vi "Autonomous Independent.vi"   [LabVIEW 2015]
doc: "This VI is called when autonomous begins, and will automatically be terminated when autonomous ends. You can carry out timed or sensor driven robot movement independently without needing to return to the caller."
uses:
  <vilib>/Rock Robotics/WPI/Utilities/WPI_GetSetVariantRefNum.vi
  <vilib>/Rock Robotics/Network Tables/NT Read String.vi
  <vilib>/Rock Robotics/Network Tables/NT Write Numeric Array.vi
  <vilib>/Rock Robotics/Network Tables/NT Read Number.vi
  <vilib>/Rock Robotics/WPI/RobotDrive/WPI_RobotDriveArcadeDrive_Standard(NoSaturation).vi
  <vilib>/Rock Robotics/WPI/RobotDrive/WPI_RobotDriveSafetyCheck.vi
panel:
  # "Be sure to right-click and choose Data Operations>>Make Current Value default if you want to save the array values with the VI"
types:
  T1 = typedef "WPI_JoystickDevRef.ctl" = cluster{"Device":T2}
  T2 = typedef "WPI_JoystickDeviceEnum.ctl" = enum16{"USB 0", "USB 1", "USB 2", "USB 3", "USB 4", "USB 5"}
  T3 = typedef "WPI_RobotDriveDevRef.ctl" = cluster{"DevStatus":errorcluster, "Motors[]":T4[], "Square Inputs":bool, "Max Output":dbl}
  T4 = typedef "WPI_MotorControlDeviceRef.ctl" = cluster{"DeviceStatus":errorcluster, "Type":T5, "PWM":cluster{"PWM Channel":T6, "DeadBand":T7}, "CAN":cluster{"Device Number":u8, "Control Mode":T8, "Semaphore":T9, "Max Vout":dbl, "TalonSRX Control Mode":T10}, "Invert":bool}
  T5 = typedef "WPI_MotorControlType.ctl" = enum16{"PWM", "CAN", "CANTalonSRX"}
  T6 = typedef "FPGA_DIOPWMChannel.ctl" = enum8{"PWM 0", "PWM 1", "PWM 2", "PWM 3", "PWM 4", "PWM 5", "PWM 6", "PWM 7", "PWM 8", "PWM 9", "PWM MXP 0", "PWM MXP 1", "PWM MXP 2", "PWM MXP 3", "PWM MXP 4", "PWM MXP 5", "PWM MXP 6", "PWM MXP 7", "PWM MXP 8", "PWM MXP 9", "Invalid"}
  T7 = typedef "WPI_PWMDeadband.ctl" = cluster{"Name":string, "maxPositivePwm":i32, "minPositivePwm":i32, "centerPwm":i32, "maxNegativePwm":i32, "minNegativePwm":i32, "angularRange":u16}
  T8 = typedef "WPI_CANJaguar_ControlMode.ctl" = enum8{"Percent VBus", "Current", "Speed", "Position", "Voltage"}
  T9 = typedef "Semaphore RefNum" = refnum<k1>
  T10 = typedef "WPI_CANTalonSRX_APIControlMode.ctl" = enum8{"Percent VBus", "Speed", "Position", "Slave", "Unchanged / Invalid", "Voltage Compensation", "Current", "Motion Profile"}
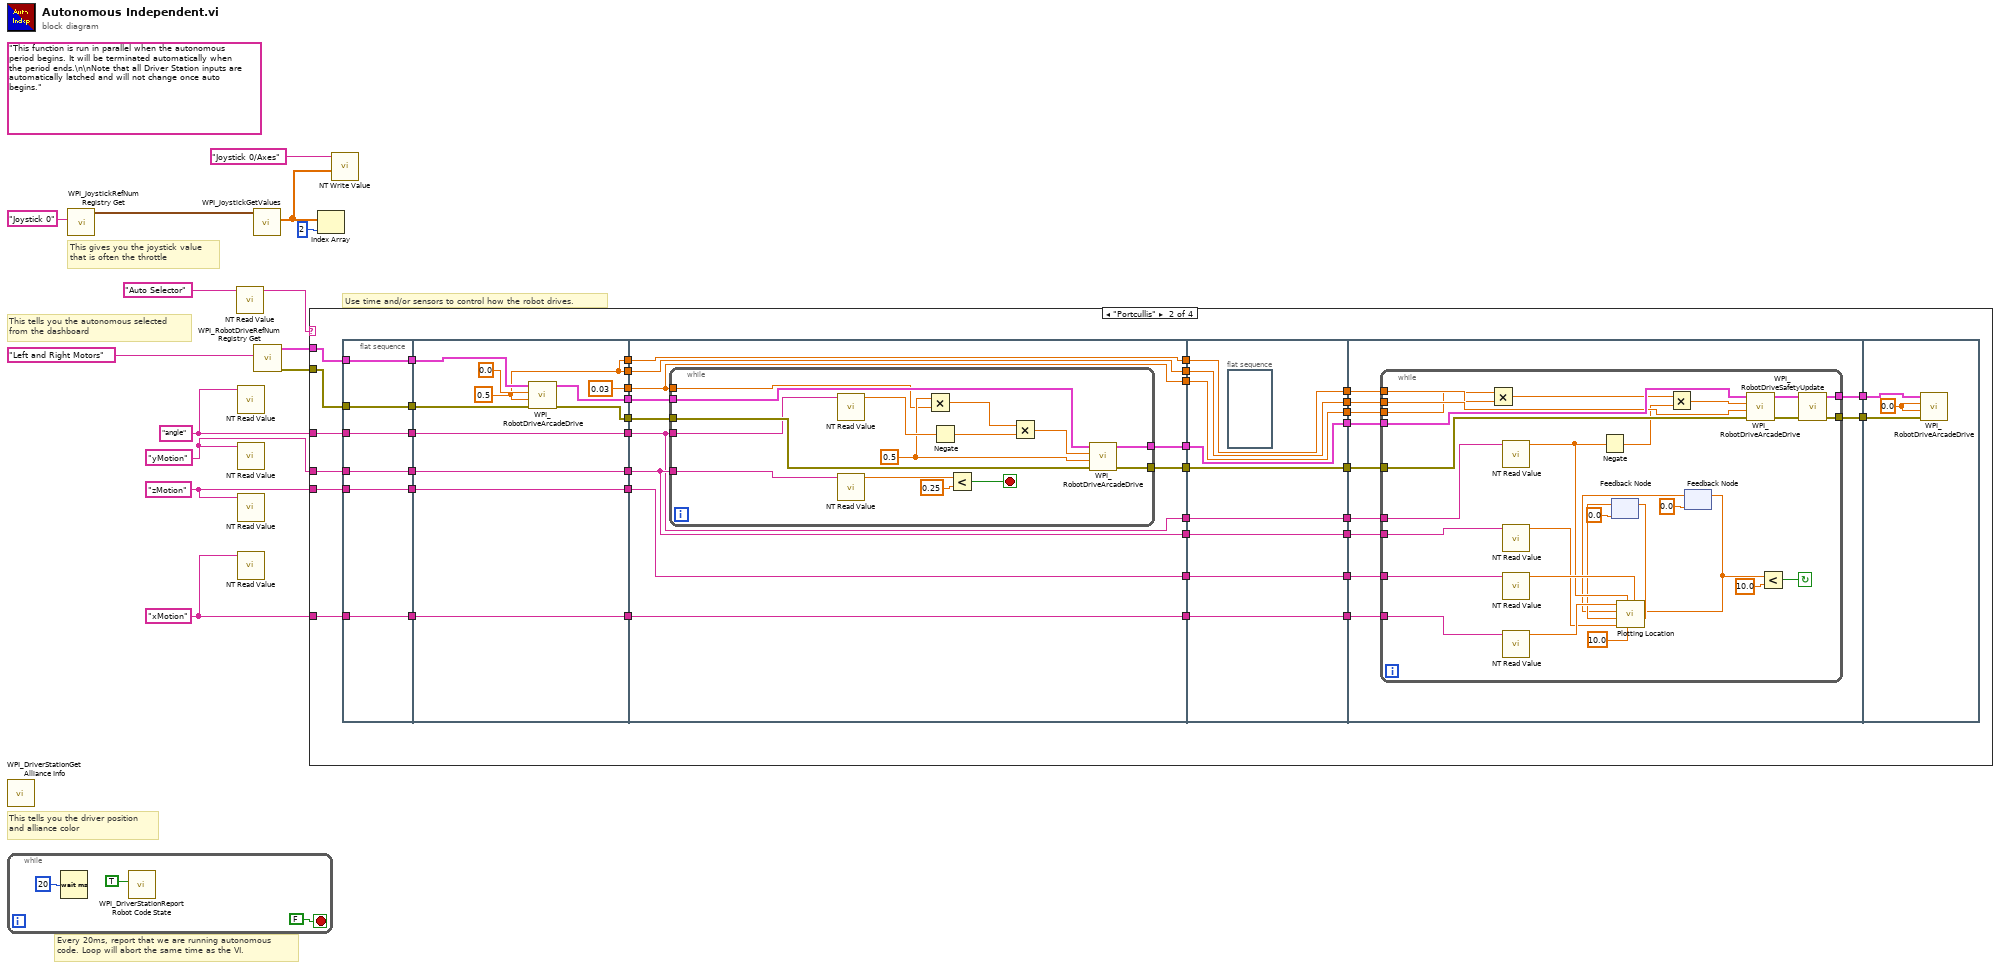
[diagram p0: block diagram]
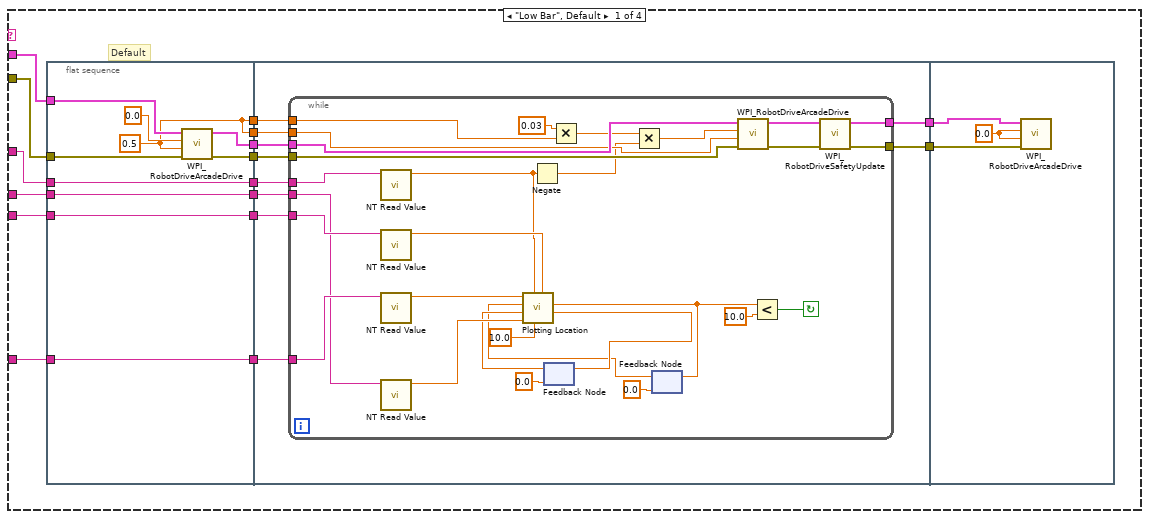
[diagram p2: hidden frame]
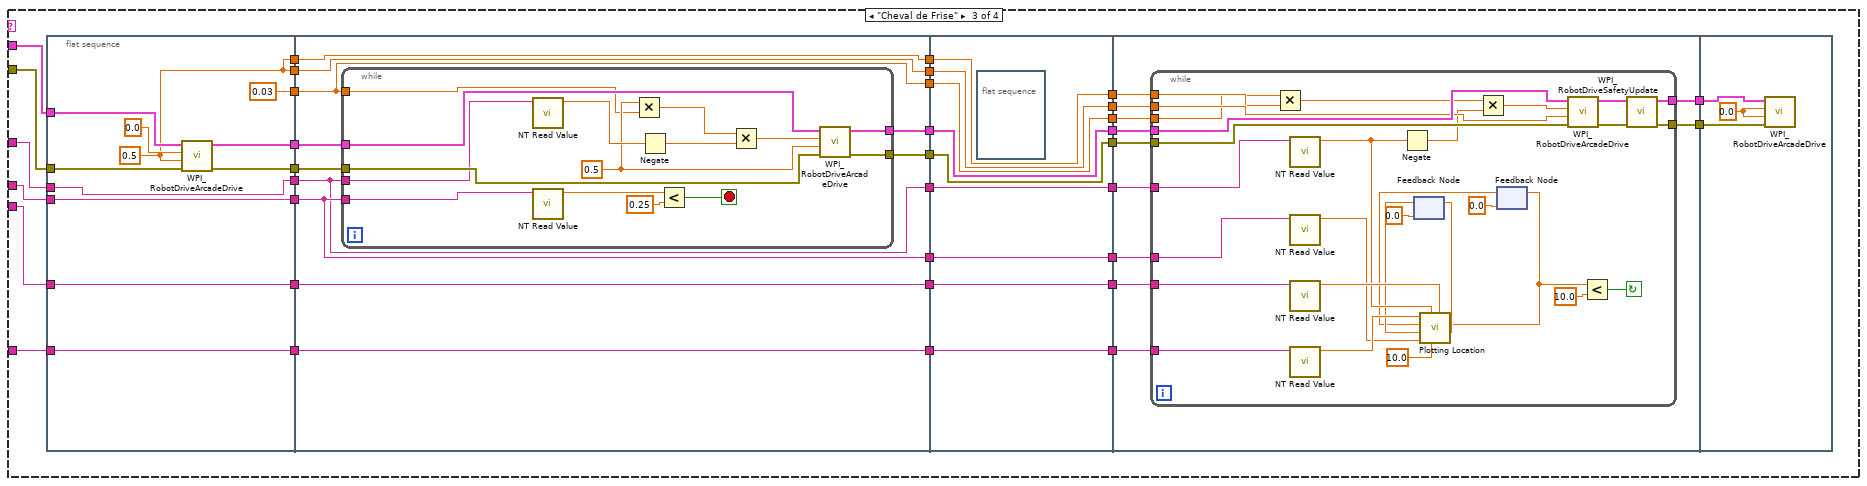
[diagram p3: hidden frame]
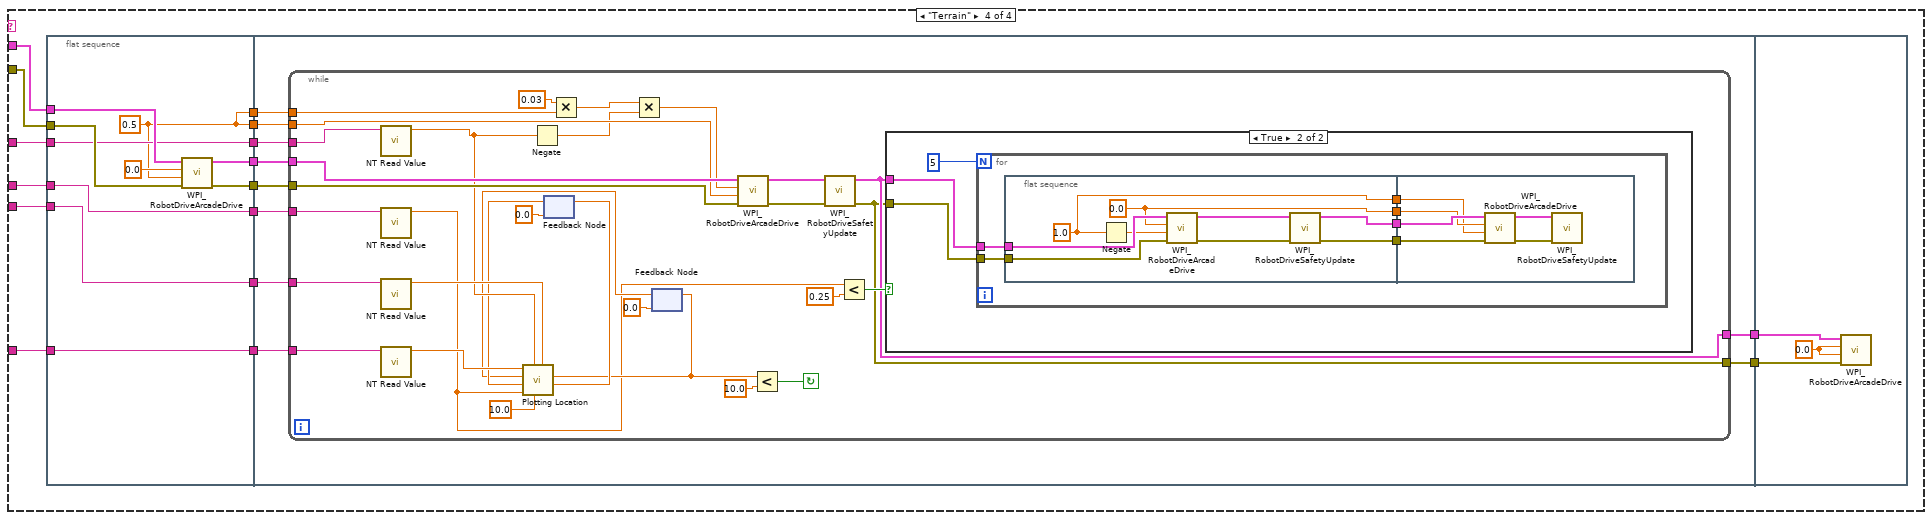
[diagram p4: hidden frame]
diagram:
  w4 = "angle" ("Name")
  w1 = "yMotion" ("Name")
  w2 = "zMotion" ("Name")
  w3 = "xMotion" ("Name")
  (unwired) "This function is run in parallel when the autonomous period begins. It will be terminated automatically when the period ends.\n\nNote that all Driver Station inputs are automatically latched and will not change once auto begins."
  # "This tells you the autonomous selected\nfrom the dashboard"
  # "Every 20ms, report that we are running autonomous\ncode. Loop will abort the same time as the VI."
  # "This gives you the joystick value\nthat is often the throttle"
  # "Use time and/or sensors to control how the robot drives."
  # "This tells you the driver position\nand alliance color"
  n1 = call <vilib>:"WPI_DriverStationGet Alliance Info.vi"() -> ()  [unwired: 12 out]
  n2 = while {
    stop <- FALSE stop-if-true
    n3 = Wait (ms)(milliseconds to wait=u32 20) -> ()  [unwired: 1 out]
    n4 = call <vilib>:"WPI_DriverStationReport Robot Code State.vi"("Autonomous"=TRUE) -> ()  [unwired: 10 in, 1 out]
  }
  n5 = call <vilib>:"WPI_JoystickRefNum Registry Get.vi"("refnum name"="Joystick 0") -> ("JoystickDevRef"=w13:T1)  [unwired: 1 in, 9 out]
  n6 = call-poly <vilib>:"NT Read Value.vi"("Name"="Auto Selector") -> ("String"=w10:string)  [unwired: 9 in, 1 out]
  n7 = call-poly <vilib>:"NT Read Value.vi"("Name"=w4) -> ()  [unwired: 9 in, 2 out]
  n8 = call-poly <vilib>:"NT Read Value.vi"("Name"=w1) -> ()  [unwired: 9 in, 2 out]
  n9 = call-poly <vilib>:"NT Read Value.vi"("Name"=w2) -> ()  [unwired: 9 in, 2 out]
  n10 = call-poly <vilib>:"NT Read Value.vi"("Name"=w3) -> ()  [unwired: 9 in, 2 out]
  n11 = call <vilib>:"WPI_JoystickGetValues.vi"("JoystickDevRef"=w13) -> ("Axes"=w9:dbl[])  [unwired: 6 in, 4 out]
  n12 = call <vilib>:"WPI_RobotDriveRefNum Registry Get.vi"("refnum name"="Left and Right Motors") -> ("error out"=w5:errorcluster, "RobotDriveDevRef"=w6:T3)  [unwired: 9 in]
  n13 = case shown="\"Portcullis\"" w10 {
    tunnel: w6 -> [w33 w124 w223 w351]
    tunnel: w5 -> [w32 w123 w222 w350]
    tunnel: w4 -> [w28 w122 w224 w349]
    tunnel: w3 -> [w26 w120 w227 w346]
    tunnel: w2 -> [w24 w121 w226 w347]
    tunnel: w1 -> [w22 w119 w225 w348]
    frame "Low Bar", Default {
      # "Default"
      n14 = flat-sequence {
        tunnel: w33 -> [w43]
        tunnel: w32 -> [w42]
        tunnel: [w40] -> w31
        tunnel: [w39] -> w30
        tunnel: [w34] -> w29
        tunnel: w28 -> [w38]
        tunnel: [w38] -> w27
        tunnel: w26 -> [w37]
        tunnel: [w37] -> w25
        tunnel: w24 -> [w36]
        tunnel: [w36] -> w23
        tunnel: w22 -> [w35]
        tunnel: [w35] -> w21
        tunnel: [w34] -> w20
        tunnel: w31 -> [w53]
        tunnel: w30 -> [w52]
        tunnel: w29 -> [w51]
        tunnel: w27 -> [w50]
        tunnel: w25 -> [w49]
        tunnel: w23 -> [w48]
        tunnel: w21 -> [w47]
        tunnel: w20 -> [w46]
        tunnel: [w45] -> w19
        tunnel: [w44] -> w18
        tunnel: w19 -> [w85]
        tunnel: w18 -> [w84]
        frame #0 {
          w34 = 0.5 ("Y axis value")
          n15 = call-poly <vilib>:"WPI_RobotDriveArcadeDrive.vi"("error in (no error)"=w42, "Y axis value"=w34, "X axis value"=0.0, "RobotDriveDevRef"=w43) -> ("error out"=w39:errorcluster, "RobotDriveDevRef"=w40:T3)  [unwired: 5 in, 1 out]
        }
        frame #1 {
          n16 = while {
            tunnel: w53 -> [w80]
            tunnel: w52 -> [w79]
            tunnel: w51 -> [w78]
            tunnel: w50 -> [w75]
            tunnel: w49 -> [w74]
            tunnel: w48 -> [w73]
            tunnel: w47 -> [w72]
            tunnel: w46 -> [w70]
            tunnel: [w55] -> w45
            tunnel: [w54] -> w44
            stop <- w63 continue-if-true
            n17 = call-poly <vilib>:"NT Read Value.vi"("Name"=w75) -> ("Numeric"=w65:dbl)  [unwired: 9 in, 1 out]
            n18 = call-poly <vilib>:"NT Read Value.vi"("Name"=w73) -> ("Numeric"=w68:dbl)  [unwired: 9 in, 1 out]
            n19 = call-poly <vilib>:"NT Read Value.vi"("Name"=w74) -> ("Numeric"=w67:dbl)  [unwired: 9 in, 1 out]
            n20 = call-poly <vilib>:"NT Read Value.vi"("Name"=w72) -> ("Numeric"=w66:dbl)  [unwired: 9 in, 1 out]
            n21 = Negate(x=w65) -> (-x=w76:dbl)
            n22 = feedback #1(0.0 ("New Y")) -> (w61:dbl)
            n23 = Multiply(x=0.03, y=w70) -> (x*y=w69:dbl)
            n24 = Multiply(x=w69, y=w76) -> (x*y=w77:dbl)
            n25 = feedback #2(0.0 ("New X")) -> (w58:dbl)
            n26 = call "Plotting Location.vi"("Z Adaption"=w68, "Refresh Rate (ms)"=10.0, "Angle"=w65, "Y-Motion"=w66, "Old Y"=w61, "Old X"=w58, "X-Motion"=w67) -> ("New Y"=w62:dbl, "New X"=w59:dbl)  [unwired: 3 in]
            n27 = feedback-in #1(w62) -> ()
            n28 = feedback-in #2(w59) -> ()
            n29 = call-poly <vilib>:"WPI_RobotDriveArcadeDrive.vi"("error in (no error)"=w79, "Y axis value"=w78, "X axis value"=w77, "RobotDriveDevRef"=w80) -> ("error out"=w81:errorcluster, "RobotDriveDevRef"=w82:T3)  [unwired: 5 in, 1 out]
            n30 = Less?(x=w59, y=10.0) -> (x < y?=w63:bool)
            n31 = call <vilib>:"WPI_RobotDriveSafetyUpdate.vi"("error in (no error)"=w81, "RobotDriveDevRef"=w82) -> ("error out"=w54:errorcluster, "RobotDriveDevRef"=w55:T3)  [unwired: 8 out]
          }
        }
        frame #2 {
          w83 = 0.0 ("X axis value")
          n32 = call-poly <vilib>:"WPI_RobotDriveArcadeDrive.vi"("error in (no error)"=w84, "Y axis value"=w83, "X axis value"=w83, "RobotDriveDevRef"=w85) -> ()  [unwired: 5 in, 3 out]
        }
      }
    }
    frame "Portcullis" {
      n33 = flat-sequence {
        tunnel: w119 -> [w127]
        tunnel: w121 -> [w128]
        tunnel: w120 -> [w129]
        tunnel: w122 -> [w130]
        tunnel: w123 -> [w131]
        tunnel: w124 -> [w132]
        tunnel: [w132] -> w91
        tunnel: [w131] -> w90
        tunnel: [w130] -> w89
        tunnel: [w129] -> w88
        tunnel: [w128] -> w87
        tunnel: [w127] -> w86
        tunnel: [w140] -> w118
        tunnel: [w139] -> w117
        tunnel: [w134] -> w116
        tunnel: [w138] -> w115
        tunnel: [w137] -> w114
        tunnel: [w136] -> w113
        tunnel: [w135] -> w112
        tunnel: [w134] -> w111
        tunnel: [0.03 ("x")] -> w93
        tunnel: w91 -> [w143]
        tunnel: w90 -> [w142]
        tunnel: w89 -> [w138]
        tunnel: w88 -> [w137]
        tunnel: w87 -> [w136]
        tunnel: w86 -> [w135]
        tunnel: w118 -> [w149]
        tunnel: w117 -> [w148]
        tunnel: [w146] -> w109
        tunnel: w116 -> [w154]
        tunnel: [w154] -> w107
        tunnel: w115 -> [w145]
        tunnel: [w145] -> w105
        tunnel: w114 -> [w153]
        tunnel: [w153] -> w103
        tunnel: w113 -> [w152]
        tunnel: [w152] -> w101
        tunnel: w112 -> [w150]
        tunnel: [w150] -> w99
        tunnel: w111 -> [w151]
        tunnel: [w151] -> w97
        tunnel: [w144] -> w94
        tunnel: w93 -> [w144]
        tunnel: [w147] -> w92
        tunnel: [w178] -> w110
        tunnel: w109 -> [w177]
        tunnel: [w177] -> w108
        tunnel: w107 -> [w176]
        tunnel: [w176] -> w106
        tunnel: w105 -> [w175]
        tunnel: [w175] -> w104
        tunnel: w103 -> [w174]
        tunnel: [w174] -> w102
        tunnel: w101 -> [w173]
        tunnel: [w173] -> w100
        tunnel: w99 -> [w172]
        tunnel: [w172] -> w98
        tunnel: w97 -> [w171]
        tunnel: [w171] -> w96
        tunnel: [w170] -> w95
        tunnel: w94 -> [w170]
        tunnel: w92 -> [w178]
        tunnel: w110 -> [w189]
        tunnel: w108 -> [w188]
        tunnel: w106 -> [w187]
        tunnel: w104 -> [w186]
        tunnel: w102 -> [w185]
        tunnel: w100 -> [w184]
        tunnel: w98 -> [w183]
        tunnel: w96 -> [w182]
        tunnel: [w181] -> w126
        tunnel: [w180] -> w125
        tunnel: w95 -> [w179]
        tunnel: w126 -> [w221]
        tunnel: w125 -> [w220]
        frame #0 {
        }
        frame #1 {
          w134 = 0.5 ("Y axis value")
          n34 = call-poly <vilib>:"WPI_RobotDriveArcadeDrive.vi"("error in (no error)"=w142, "Y axis value"=w134, "X axis value"=0.0, "RobotDriveDevRef"=w143) -> ("error out"=w139:errorcluster, "RobotDriveDevRef"=w140:T3)  [unwired: 5 in, 1 out]
        }
        frame #2 {
          n35 = while {
            tunnel: w150 -> [w166]
            tunnel: w149 -> [w165]
            tunnel: w148 -> [w164]
            tunnel: [w163] -> w147
            tunnel: [w162] -> w146
            tunnel: w145 -> [w161]
            tunnel: w144 -> [w156]
            stop <- w167 stop-if-true
            w157 = 0.5 ("Y axis value")
            n36 = call-poly <vilib>:"NT Read Value.vi"("Name"=w161) -> ("Numeric"=w158:dbl)  [unwired: 9 in, 1 out]
            n37 = call-poly <vilib>:"NT Read Value.vi"("Name"=w166) -> ("Numeric"=w169:dbl)  [unwired: 9 in, 1 out]
            n38 = Multiply(x=w157, y=w156) -> (x*y=w159:dbl)
            n39 = Negate(x=w158) -> (-x=w160:dbl)
            n40 = Less?(x=w169, y=0.25) -> (x < y?=w167:bool)
            n41 = Multiply(x=w159, y=w160) -> (x*y=w155:dbl)
            n42 = call-poly <vilib>:"WPI_RobotDriveArcadeDrive.vi"("error in (no error)"=w164, "Y axis value"=w157, "X axis value"=w155, "RobotDriveDevRef"=w165) -> ("error out"=w162:errorcluster, "RobotDriveDevRef"=w163:T3)  [unwired: 5 in, 1 out]
          }
        }
        frame #3 {
          n43 = flat-sequence {
            frame #0 {
            }
          }
        }
        frame #4 {
          n44 = while {
            tunnel: w189 -> [w216]
            tunnel: w188 -> [w215]
            tunnel: w187 -> [w214]
            tunnel: w186 -> [w211]
            tunnel: w185 -> [w210]
            tunnel: w184 -> [w209]
            tunnel: w183 -> [w208]
            tunnel: w182 -> [w207]
            tunnel: [w192] -> w181
            tunnel: [w191] -> w180
            tunnel: w179 -> [w190]
            stop <- w200 continue-if-true
            n45 = Multiply(x=w190, y=w207) -> (x*y=w206:dbl)
            n46 = call-poly <vilib>:"NT Read Value.vi"("Name"=w211) -> ("Numeric"=w202:dbl)  [unwired: 9 in, 1 out]
            n47 = call-poly <vilib>:"NT Read Value.vi"("Name"=w208) -> ("Numeric"=w203:dbl)  [unwired: 9 in, 1 out]
            n48 = call-poly <vilib>:"NT Read Value.vi"("Name"=w209) -> ("Numeric"=w205:dbl)  [unwired: 9 in, 1 out]
            n49 = call-poly <vilib>:"NT Read Value.vi"("Name"=w210) -> ("Numeric"=w204:dbl)  [unwired: 9 in, 1 out]
            n50 = Negate(x=w202) -> (-x=w212:dbl)
            n51 = feedback #3(0.0 ("New Y")) -> (w198:dbl)
            n52 = Multiply(x=w206, y=w212) -> (x*y=w213:dbl)
            n53 = feedback #4(0.0 ("New X")) -> (w195:dbl)
            n54 = call "Plotting Location.vi"("Z Adaption"=w205, "Refresh Rate (ms)"=10.0, "Angle"=w202, "Y-Motion"=w203, "Old Y"=w198, "Old X"=w195, "X-Motion"=w204) -> ("New Y"=w199:dbl, "New X"=w196:dbl)  [unwired: 3 in]
            n55 = feedback-in #3(w199) -> ()
            n56 = feedback-in #4(w196) -> ()
            n57 = call-poly <vilib>:"WPI_RobotDriveArcadeDrive.vi"("error in (no error)"=w215, "Y axis value"=w214, "X axis value"=w213, "RobotDriveDevRef"=w216) -> ("error out"=w217:errorcluster, "RobotDriveDevRef"=w218:T3)  [unwired: 5 in, 1 out]
            n58 = Less?(x=w196, y=10.0) -> (x < y?=w200:bool)
            n59 = call <vilib>:"WPI_RobotDriveSafetyUpdate.vi"("error in (no error)"=w217, "RobotDriveDevRef"=w218) -> ("error out"=w191:errorcluster, "RobotDriveDevRef"=w192:T3)  [unwired: 8 out]
          }
        }
        frame #5 {
          w219 = 0.0 ("X axis value")
          n60 = call-poly <vilib>:"WPI_RobotDriveArcadeDrive.vi"("error in (no error)"=w220, "Y axis value"=w219, "X axis value"=w219, "RobotDriveDevRef"=w221) -> ()  [unwired: 5 in, 3 out]
        }
      }
    }
    frame "Cheval de Frise" {
      n61 = flat-sequence {
        tunnel: w223 -> [w267]
        tunnel: w222 -> [w266]
        tunnel: [w264] -> w256
        tunnel: [w263] -> w255
        tunnel: [w258] -> w254
        tunnel: w224 -> [w262]
        tunnel: [w262] -> w253
        tunnel: w227 -> [w261]
        tunnel: [w261] -> w252
        tunnel: w226 -> [w260]
        tunnel: [w260] -> w251
        tunnel: w225 -> [w259]
        tunnel: [w259] -> w250
        tunnel: [w258] -> w249
        tunnel: [0.03 ("x")] -> w248
        tunnel: w256 -> [w273]
        tunnel: w255 -> [w272]
        tunnel: [w270] -> w247
        tunnel: w254 -> [w278]
        tunnel: [w278] -> w246
        tunnel: w253 -> [w269]
        tunnel: [w269] -> w245
        tunnel: w252 -> [w277]
        tunnel: [w277] -> w244
        tunnel: w251 -> [w276]
        tunnel: [w276] -> w243
        tunnel: w250 -> [w274]
        tunnel: [w274] -> w242
        tunnel: w249 -> [w275]
        tunnel: [w275] -> w241
        tunnel: [w268] -> w240
        tunnel: w248 -> [w268]
        tunnel: [w271] -> w239
        tunnel: [w302] -> w238
        tunnel: w247 -> [w301]
        tunnel: [w301] -> w237
        tunnel: w246 -> [w300]
        tunnel: [w300] -> w236
        tunnel: w245 -> [w299]
        tunnel: [w299] -> w235
        tunnel: w244 -> [w298]
        tunnel: [w298] -> w234
        tunnel: w243 -> [w297]
        tunnel: [w297] -> w233
        tunnel: w242 -> [w296]
        tunnel: [w296] -> w232
        tunnel: w241 -> [w295]
        tunnel: [w295] -> w231
        tunnel: [w294] -> w230
        tunnel: w240 -> [w294]
        tunnel: w239 -> [w302]
        tunnel: w238 -> [w313]
        tunnel: w237 -> [w312]
        tunnel: w236 -> [w311]
        tunnel: w235 -> [w310]
        tunnel: w234 -> [w309]
        tunnel: w233 -> [w308]
        tunnel: w232 -> [w307]
        tunnel: w231 -> [w306]
        tunnel: [w305] -> w229
        tunnel: [w304] -> w228
        tunnel: w230 -> [w303]
        tunnel: w229 -> [w345]
        tunnel: w228 -> [w344]
        frame #0 {
          w258 = 0.5 ("Y axis value")
          n62 = call-poly <vilib>:"WPI_RobotDriveArcadeDrive.vi"("error in (no error)"=w266, "Y axis value"=w258, "X axis value"=0.0, "RobotDriveDevRef"=w267) -> ("error out"=w263:errorcluster, "RobotDriveDevRef"=w264:T3)  [unwired: 5 in, 1 out]
        }
        frame #1 {
          n63 = while {
            tunnel: w274 -> [w290]
            tunnel: w273 -> [w289]
            tunnel: w272 -> [w288]
            tunnel: [w287] -> w271
            tunnel: [w286] -> w270
            tunnel: w269 -> [w285]
            tunnel: w268 -> [w280]
            stop <- w291 stop-if-true
            w281 = 0.5 ("Y axis value")
            n64 = call-poly <vilib>:"NT Read Value.vi"("Name"=w285) -> ("Numeric"=w282:dbl)  [unwired: 9 in, 1 out]
            n65 = call-poly <vilib>:"NT Read Value.vi"("Name"=w290) -> ("Numeric"=w293:dbl)  [unwired: 9 in, 1 out]
            n66 = Multiply(x=w281, y=w280) -> (x*y=w283:dbl)
            n67 = Negate(x=w282) -> (-x=w284:dbl)
            n68 = Less?(x=w293, y=0.25) -> (x < y?=w291:bool)
            n69 = Multiply(x=w283, y=w284) -> (x*y=w279:dbl)
            n70 = call-poly <vilib>:"WPI_RobotDriveArcadeDrive.vi"("error in (no error)"=w288, "Y axis value"=w281, "X axis value"=w279, "RobotDriveDevRef"=w289) -> ("error out"=w286:errorcluster, "RobotDriveDevRef"=w287:T3)  [unwired: 5 in, 1 out]
          }
        }
        frame #2 {
          n71 = flat-sequence {
            frame #0 {
            }
          }
        }
        frame #3 {
          n72 = while {
            tunnel: w313 -> [w340]
            tunnel: w312 -> [w339]
            tunnel: w311 -> [w338]
            tunnel: w310 -> [w335]
            tunnel: w309 -> [w334]
            tunnel: w308 -> [w333]
            tunnel: w307 -> [w332]
            tunnel: w306 -> [w331]
            tunnel: [w316] -> w305
            tunnel: [w315] -> w304
            tunnel: w303 -> [w314]
            stop <- w324 continue-if-true
            n73 = Multiply(x=w314, y=w331) -> (x*y=w330:dbl)
            n74 = call-poly <vilib>:"NT Read Value.vi"("Name"=w335) -> ("Numeric"=w326:dbl)  [unwired: 9 in, 1 out]
            n75 = call-poly <vilib>:"NT Read Value.vi"("Name"=w332) -> ("Numeric"=w327:dbl)  [unwired: 9 in, 1 out]
            n76 = call-poly <vilib>:"NT Read Value.vi"("Name"=w333) -> ("Numeric"=w329:dbl)  [unwired: 9 in, 1 out]
            n77 = call-poly <vilib>:"NT Read Value.vi"("Name"=w334) -> ("Numeric"=w328:dbl)  [unwired: 9 in, 1 out]
            n78 = Negate(x=w326) -> (-x=w336:dbl)
            n79 = feedback #5(0.0 ("New Y")) -> (w322:dbl)
            n80 = Multiply(x=w330, y=w336) -> (x*y=w337:dbl)
            n81 = feedback #6(0.0 ("New X")) -> (w319:dbl)
            n82 = call "Plotting Location.vi"("Z Adaption"=w329, "Refresh Rate (ms)"=10.0, "Angle"=w326, "Y-Motion"=w327, "Old Y"=w322, "Old X"=w319, "X-Motion"=w328) -> ("New Y"=w323:dbl, "New X"=w320:dbl)  [unwired: 3 in]
            n83 = feedback-in #5(w323) -> ()
            n84 = feedback-in #6(w320) -> ()
            n85 = call-poly <vilib>:"WPI_RobotDriveArcadeDrive.vi"("error in (no error)"=w339, "Y axis value"=w338, "X axis value"=w337, "RobotDriveDevRef"=w340) -> ("error out"=w341:errorcluster, "RobotDriveDevRef"=w342:T3)  [unwired: 5 in, 1 out]
            n86 = Less?(x=w320, y=10.0) -> (x < y?=w324:bool)
            n87 = call <vilib>:"WPI_RobotDriveSafetyUpdate.vi"("error in (no error)"=w341, "RobotDriveDevRef"=w342) -> ("error out"=w315:errorcluster, "RobotDriveDevRef"=w316:T3)  [unwired: 8 out]
          }
        }
        frame #4 {
          w343 = 0.0 ("X axis value")
          n88 = call-poly <vilib>:"WPI_RobotDriveArcadeDrive.vi"("error in (no error)"=w344, "Y axis value"=w343, "X axis value"=w343, "RobotDriveDevRef"=w345) -> ()  [unwired: 5 in, 3 out]
        }
      }
    }
    frame "Terrain" {
      n89 = flat-sequence {
        tunnel: w351 -> [w371]
        tunnel: w350 -> [w370]
        tunnel: [w368] -> w361
        tunnel: [w367] -> w360
        tunnel: [w362] -> w359
        tunnel: w349 -> [w366]
        tunnel: [w366] -> w358
        tunnel: w346 -> [w365]
        tunnel: [w365] -> w357
        tunnel: w347 -> [w364]
        tunnel: [w364] -> w356
        tunnel: w348 -> [w363]
        tunnel: [w363] -> w355
        tunnel: [w362] -> w354
        tunnel: w361 -> [w381]
        tunnel: w360 -> [w380]
        tunnel: w359 -> [w379]
        tunnel: w358 -> [w378]
        tunnel: w357 -> [w377]
        tunnel: w356 -> [w376]
        tunnel: w355 -> [w375]
        tunnel: w354 -> [w374]
        tunnel: [w373] -> w353
        tunnel: [w372] -> w352
        tunnel: w353 -> [w439]
        tunnel: w352 -> [w438]
        frame #0 {
          w362 = 0.5 ("Y axis value")
          n90 = call-poly <vilib>:"WPI_RobotDriveArcadeDrive.vi"("error in (no error)"=w370, "Y axis value"=w362, "X axis value"=0.0, "RobotDriveDevRef"=w371) -> ("error out"=w367:errorcluster, "RobotDriveDevRef"=w368:T3)  [unwired: 5 in, 1 out]
        }
        frame #1 {
          n91 = while {
            tunnel: w381 -> [w410]
            tunnel: w380 -> [w409]
            tunnel: w379 -> [w408]
            tunnel: w378 -> [w405]
            tunnel: w377 -> [w404]
            tunnel: w376 -> [w403]
            tunnel: w375 -> [w402]
            tunnel: w374 -> [w400]
            tunnel: [w383] -> w373
            tunnel: [w382] -> w372
            stop <- w394 continue-if-true
            n92 = call-poly <vilib>:"NT Read Value.vi"("Name"=w405) -> ("Numeric"=w396:dbl)  [unwired: 9 in, 1 out]
            n93 = call-poly <vilib>:"NT Read Value.vi"("Name"=w402) -> ("Numeric"=w386:dbl)  [unwired: 9 in, 1 out]
            n94 = call-poly <vilib>:"NT Read Value.vi"("Name"=w403) -> ("Numeric"=w398:dbl)  [unwired: 9 in, 1 out]
            n95 = call-poly <vilib>:"NT Read Value.vi"("Name"=w404) -> ("Numeric"=w397:dbl)  [unwired: 9 in, 1 out]
            n96 = Negate(x=w396) -> (-x=w406:dbl)
            n97 = feedback #7(0.0 ("New Y")) -> (w392:dbl)
            n98 = Multiply(x=0.03, y=w400) -> (x*y=w399:dbl)
            n99 = Multiply(x=w399, y=w406) -> (x*y=w407:dbl)
            n100 = feedback #8(0.0 ("New X")) -> (w389:dbl)
            n101 = call "Plotting Location.vi"("Z Adaption"=w398, "Refresh Rate (ms)"=10.0, "Angle"=w396, "Y-Motion"=w386, "Old Y"=w392, "Old X"=w389, "X-Motion"=w397) -> ("New Y"=w393:dbl, "New X"=w390:dbl)  [unwired: 3 in]
            n102 = feedback-in #7(w393) -> ()
            n103 = feedback-in #8(w390) -> ()
            n104 = call-poly <vilib>:"WPI_RobotDriveArcadeDrive.vi"("error in (no error)"=w409, "Y axis value"=w408, "X axis value"=w407, "RobotDriveDevRef"=w410) -> ("error out"=w411:errorcluster, "RobotDriveDevRef"=w412:T3)  [unwired: 5 in, 1 out]
            n105 = Less?(x=w390, y=10.0) -> (x < y?=w394:bool)
            n106 = call <vilib>:"WPI_RobotDriveSafetyUpdate.vi"("error in (no error)"=w411, "RobotDriveDevRef"=w412) -> ("error out"=w382:errorcluster, "RobotDriveDevRef"=w383:T3)  [unwired: 8 out]
            n107 = Less?(x=w386, y=0.25) -> (x < y?=w385:bool)
            n108 = case shown="True" w385 {
              tunnel: w383 -> [_ w414]
              tunnel: w382 -> [_ w413]
              frame False {
              }
              frame True {
                n109 = for {
                  N: 5 -> [_]
                  tunnel: w414 -> [w421]
                  tunnel: w413 -> [w420]
                  n110 = flat-sequence {
                    tunnel: w421 -> [w430]
                    tunnel: w420 -> [w429]
                    tunnel: [w427] -> w419
                    tunnel: [w426] -> w418
                    tunnel: [w424] -> w417
                    tunnel: [w423] -> w416
                    tunnel: w419 -> [w436]
                    tunnel: w418 -> [w435]
                    tunnel: w417 -> [w432]
                    tunnel: w416 -> [w431]
                    frame #0 {
                      w423 = 1.0 ("X axis value")
                      w424 = 0.0 ("X axis value")
                      n111 = Negate(x=w423) -> (-x=w422:dbl)
                      n112 = call-poly <vilib>:"WPI_RobotDriveArcadeDrive.vi"("error in (no error)"=w429, "Y axis value"=w422, "X axis value"=w424, "RobotDriveDevRef"=w430) -> ("error out"=w425:errorcluster, "RobotDriveDevRef"=w428:T3)  [unwired: 5 in, 1 out]
                      n113 = call <vilib>:"WPI_RobotDriveSafetyUpdate.vi"("error in (no error)"=w425, "RobotDriveDevRef"=w428) -> ("error out"=w426:errorcluster, "RobotDriveDevRef"=w427:T3)  [unwired: 8 out]
                    }
                    frame #1 {
                      n114 = call-poly <vilib>:"WPI_RobotDriveArcadeDrive.vi"("error in (no error)"=w435, "Y axis value"=w431, "X axis value"=w432, "RobotDriveDevRef"=w436) -> ("error out"=w433:errorcluster, "RobotDriveDevRef"=w434:T3)  [unwired: 5 in, 1 out]
                      n115 = call <vilib>:"WPI_RobotDriveSafetyUpdate.vi"("error in (no error)"=w433, "RobotDriveDevRef"=w434) -> ()  [unwired: 10 out]
                    }
                  }
                }
              }
            }
          }
        }
        frame #2 {
          w437 = 0.0 ("X axis value")
          n116 = call-poly <vilib>:"WPI_RobotDriveArcadeDrive.vi"("error in (no error)"=w438, "Y axis value"=w437, "X axis value"=w437, "RobotDriveDevRef"=w439) -> ()  [unwired: 5 in, 3 out]
        }
      }
    }
  }
  n117 = Index Array(array=w9, index=2) -> ()  [unwired: 1 out]
  n118 = call-poly <vilib>:"NT Write Value.vi"("Numeric Array"=w9, "Name"="Joystick 0/Axes") -> ()  [unwired: 9 in, 1 out]
